vi "Enable stage.vi"(8 "error in (no error)":errorcluster, 11 "Ref in":i32) -> (0 "error out":errorcluster, 3 "reference (out)":i32)   [LabVIEW 2011]
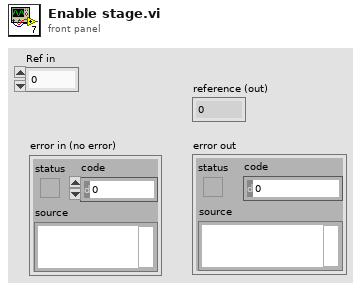
[diagram p1: front panel]
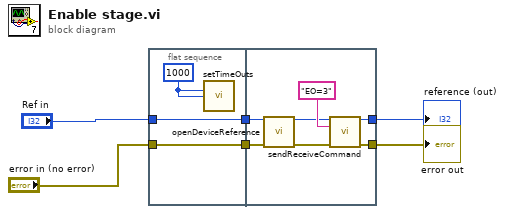
[diagram p0: block diagram]
diagram:
  n1 = flat-sequence {
    tunnel: "Ref in" -> [w8]
    tunnel: [w8] -> w6
    tunnel: "error in (no error)" -> [w7]
    tunnel: [w7] -> w5
    tunnel: w6 -> [w16]
    tunnel: w5 -> [w15]
    tunnel: [w13] -> w3
    tunnel: [w12] -> w4
    frame #0 {
      w9 = 1000 ("read_timeout")
      n2 = call "setTimeOuts.vi"("read_timeout (ms)"=w9, "write_timeout (ms)"=w9) -> ()  [unwired: 13 in, 1 out]
    }
    frame #1 {
      n3 = call "openDeviceReference.vi"("deviceIndex"=w16, "error in (no error)"=w15) -> ("reference"=w11:i32, "error out"=w10:errorcluster)  [unwired: 12 in]
      n4 = call "sendReceiveCommand.vi"("reference (in)"=w11, "write_string"="EO=3" ("raw_cmd 2"), "error in (no error)"=w10) -> ("reference (out)"=w13:i32, "error out"=w12:errorcluster)  [unwired: 10 in, 1 out]
    }
  }
  "error out" <- w4
  "reference (out)" <- w3
